vi "UserMgr-Window.vi"(7 "PwdMgr":refnum<class "PwdMgr.lvclass">, 8 "error in":errorcluster) -> (0 "error out":errorcluster)   [LabVIEW 2020, in "Login-UI.lvlib"]
uses:
  Login-UI.lvlib
  PwdMgr/PwdMgr.lvclass
  _Typedef/User-Info.ctl
  _Typedef/User-Role.ctl
  2fbc59fa-d6e3-46c3-98fb-aa3f40a50569.vi
  b49018c0-b0cc-4a1e-8c0a-6a6f7b5dc366.vi
  <userlib>/NEVSTOP-Programming-Palette/Configuration/ClusterCfgTable/Parse CfgTable(with DataName).vi
panel:
  in  "Table":i32(listbox)
  in  "编辑":bool
  in  "添加":bool
  in  "删除":bool
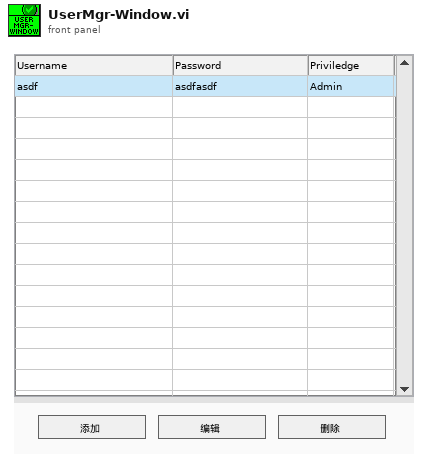
[diagram p1: front panel]
types:
  T1 = typedef "Login-UI.lvlib/User-Info.ctl" = cluster{"UserName":string, "Password":string, "Role":T2}
  T2 = typedef "Login-UI.lvlib/User-Role.ctl" = enum16{"INVALID", "Operator", "Engineer", "Admin", "Anonymous"}
  T3 = enum32{"Invalid", "Standard", "Closed", "Hidden", "Minimized", "Maximized"}
  T4 = enum32{"invalid app kind", "Development System", "Run Time System", "Student Edition", "Embedded LabVIEW", "Evaluation", "Custom"}
  T5 = cluster{"Core":cluster{"Current VI Reference":refnum<vi>, "Close Panel on Exit?":bool}, "Your Boolean data":bool, "Your string data":string, "Table Ref":refnum<vi>}
  T6 = cluster{"Current VI Reference":refnum<vi>, "Close Panel on Exit?":bool}
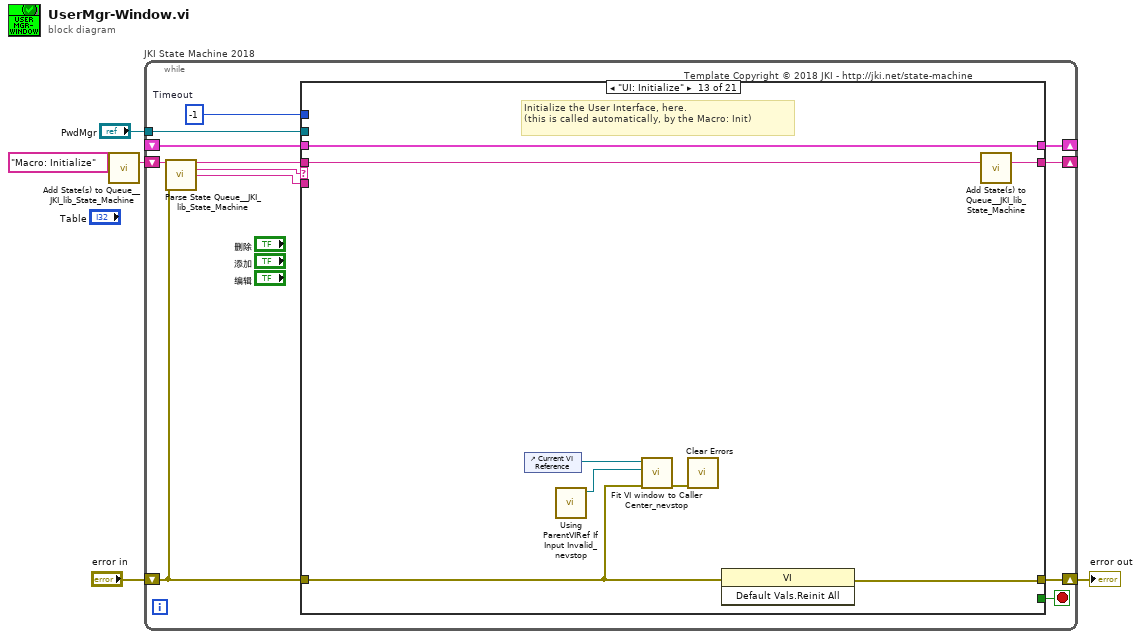
[diagram p0: block diagram]
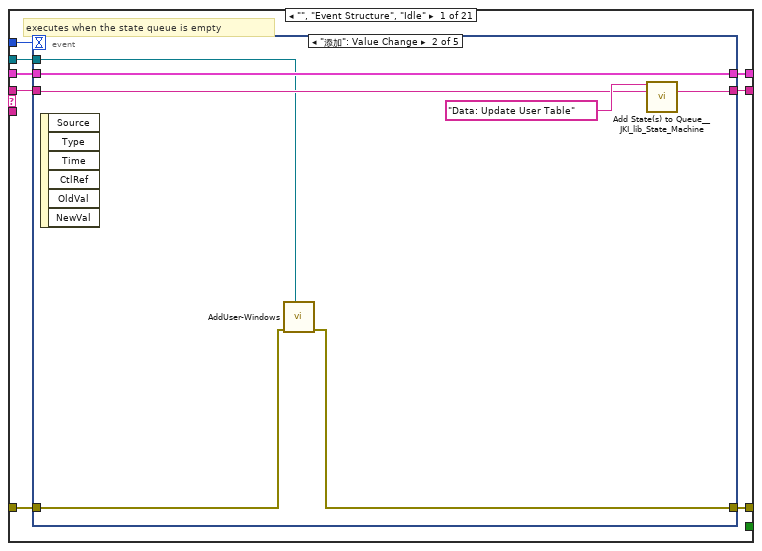
[diagram p2: hidden frame]
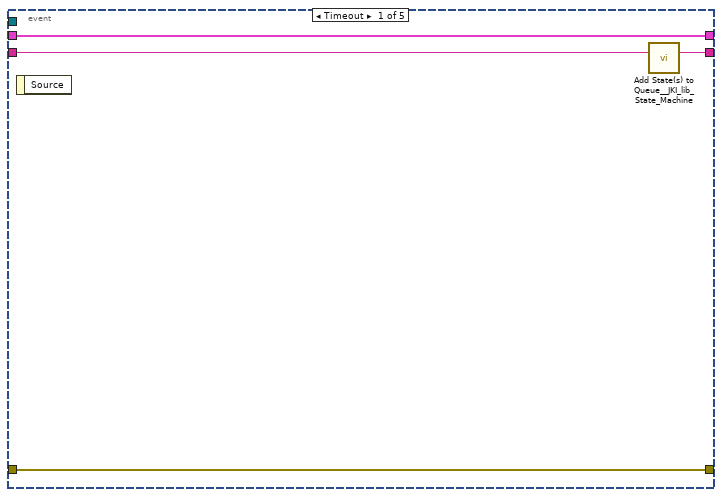
[diagram p3: hidden frame]
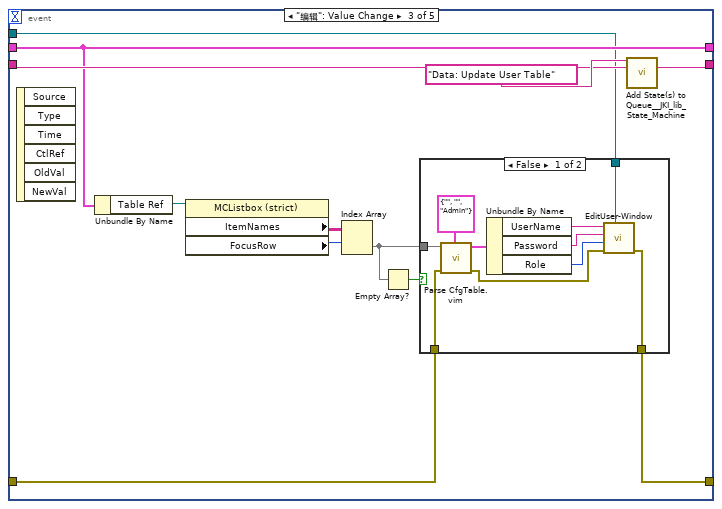
[diagram p4: hidden frame]
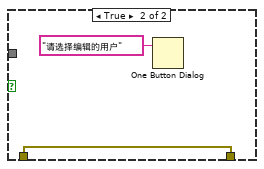
[diagram p5: hidden frame]
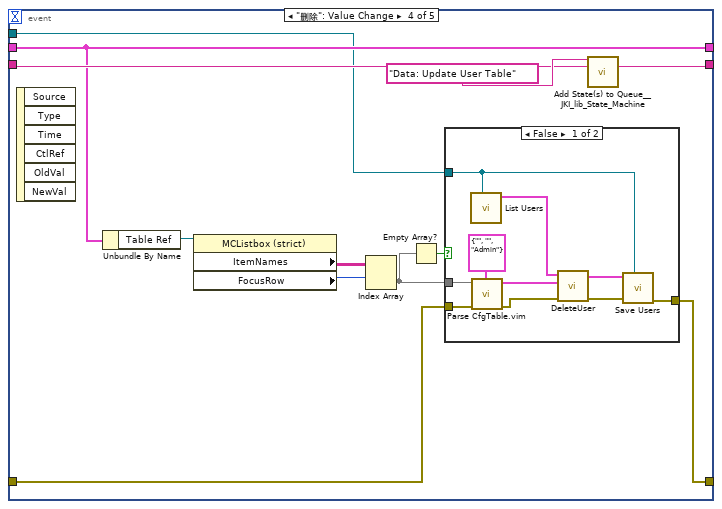
[diagram p6: hidden frame]
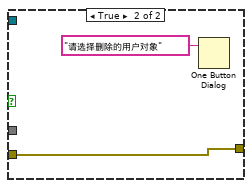
[diagram p7: hidden frame]
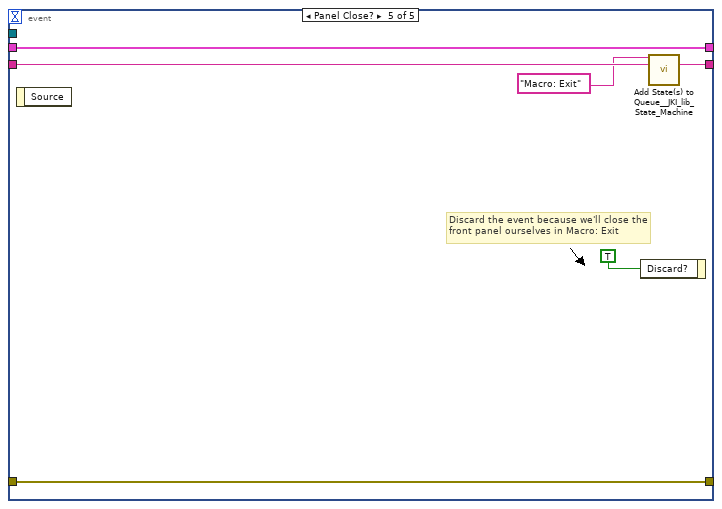
[diagram p8: hidden frame]
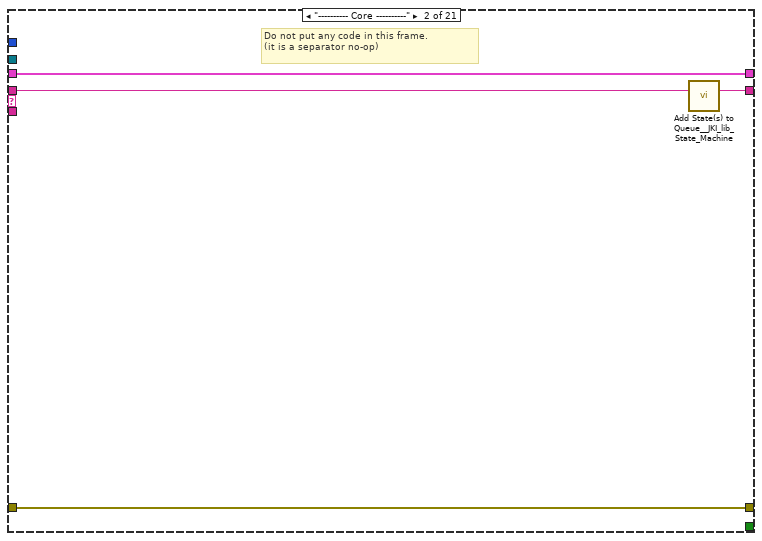
[diagram p9: hidden frame]
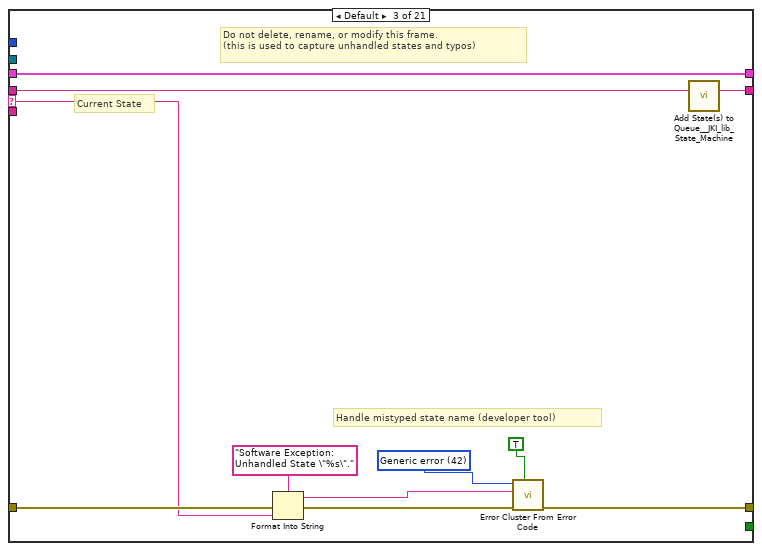
[diagram p10: hidden frame]
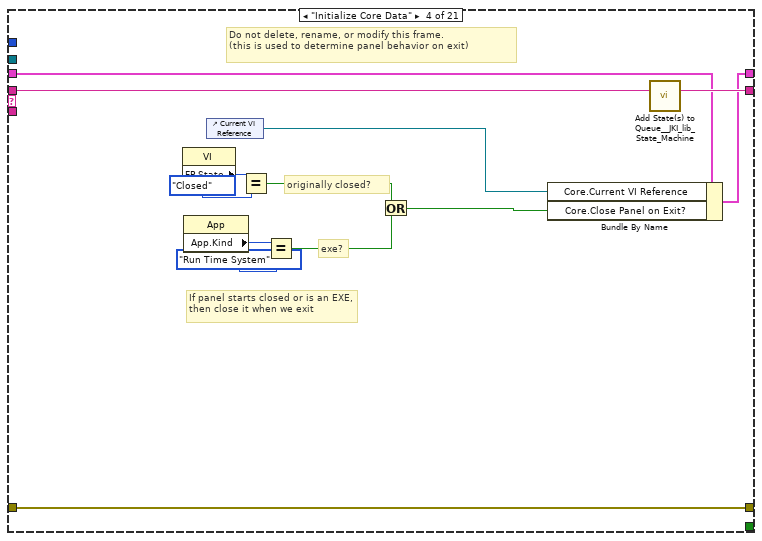
[diagram p11: hidden frame]
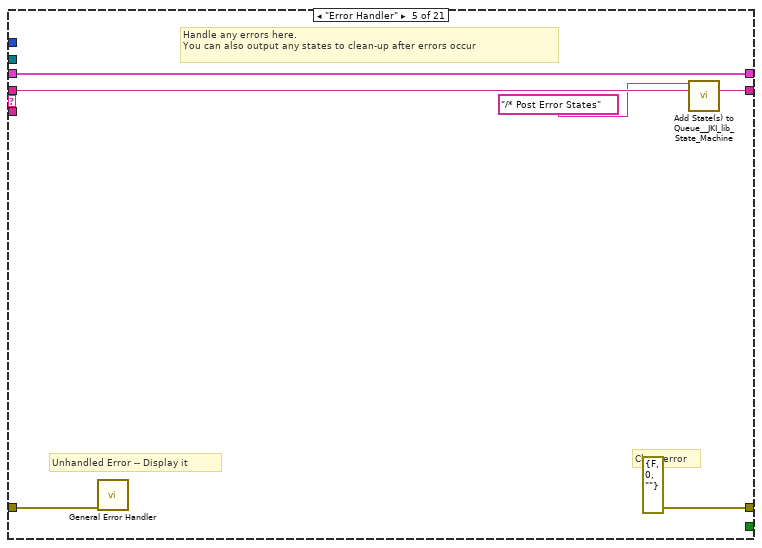
[diagram p12: hidden frame]
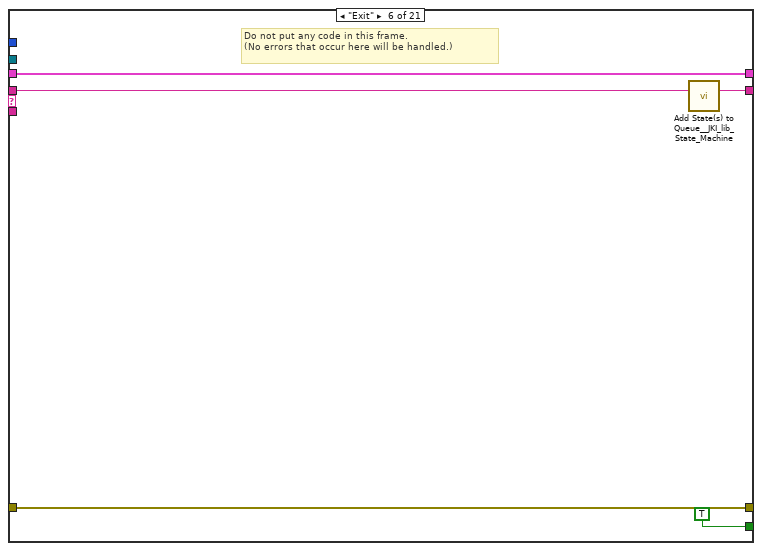
[diagram p13: hidden frame]
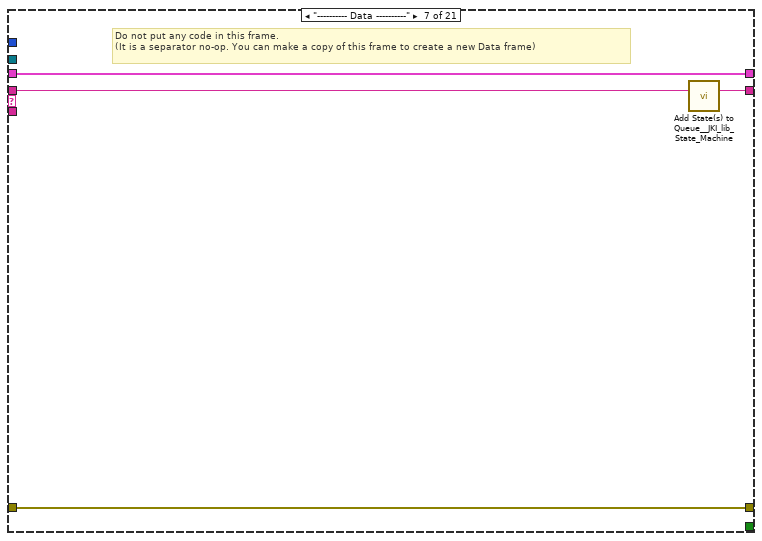
[diagram p14: hidden frame]
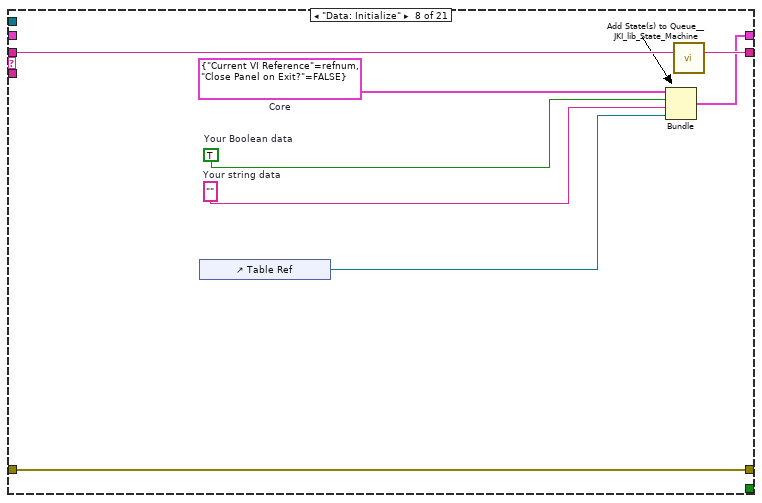
[diagram p15: hidden frame]
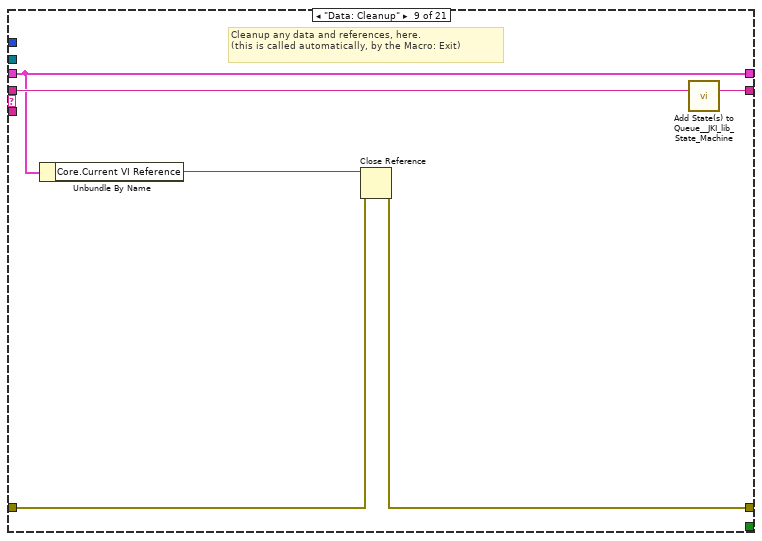
[diagram p16: hidden frame]
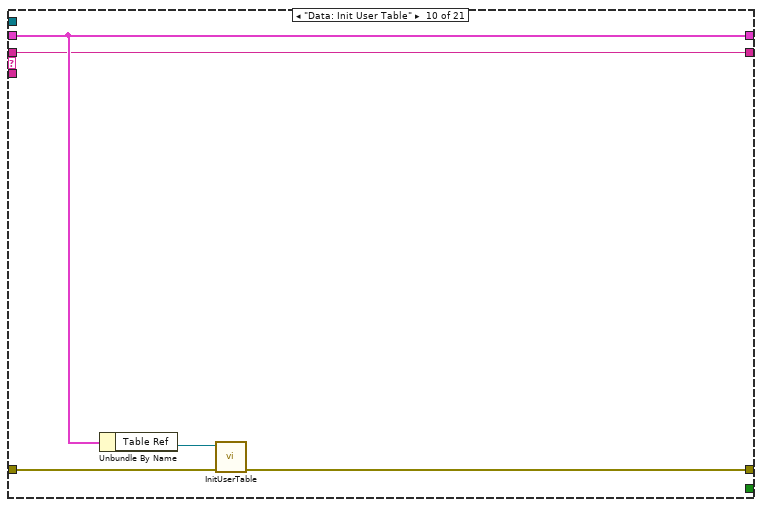
[diagram p17: hidden frame]
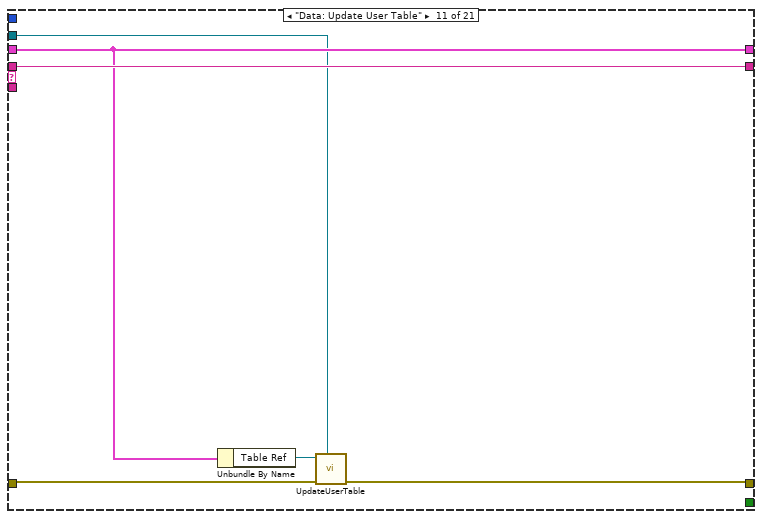
[diagram p18: hidden frame]
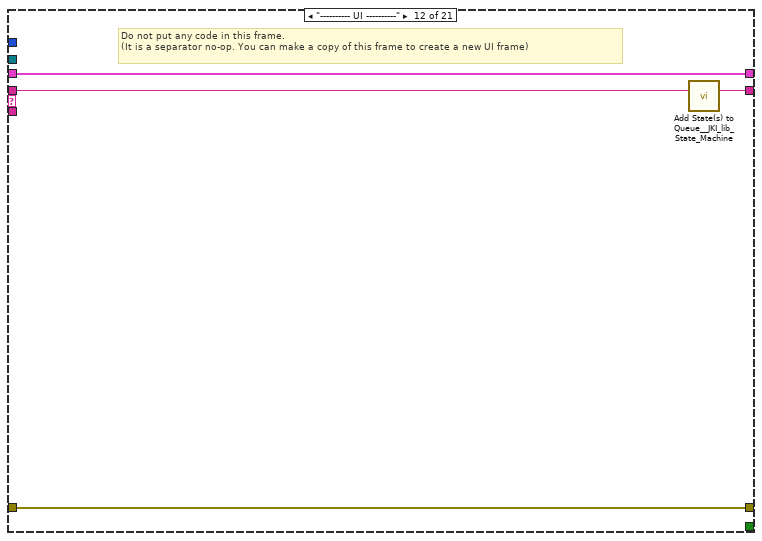
[diagram p19: hidden frame]
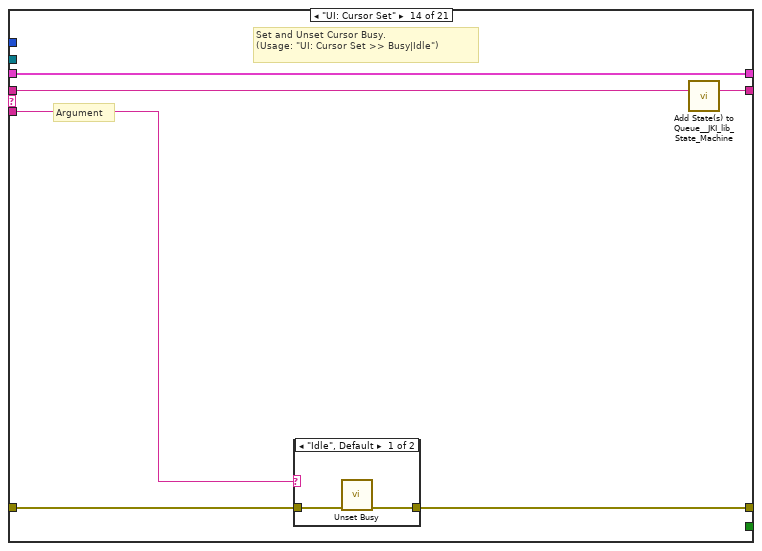
[diagram p20: hidden frame]
diagram:
  n1 = call <vilib>:"Add State(s) to Queue__JKI_lib_State_Machine.vi"("State(s) in (\"\")"="Macro: Initialize") -> ("States Out"=w5:string)  [unwired: 14 in]
  n2 = while "JKI State Machine 2018" {
    shift-right: [w10] -> _
    shift-left: _ -> [w9]
    shift-right: [w13] -> w2
    shift-left: "error in" -> [w7]
    shift-right: [w12] -> _
    shift-left: w5 -> [w14]
    tunnel: "PwdMgr" -> [w6]
    stop <- w11 stop-if-true
    w8 = -1  # Timeout
    # "Template Copyright © 2018 JKI - http://jki.net/state-machine"
    n3 = call <vilib>:"Parse State Queue__JKI_lib_State_Machine.vi"("State Queue"=w14, "Error In (no error)"=w7) -> ("Remaining States"=w16:string, "Current State"=w17:string, "Arguments"=w15:string)  [unwired: 11 in]
    n4 = case shown="\"UI: Initialize\"" w17 {
      selector: w17 -> [_ _ w95 _ _ _ _ _ _ _ _ _ _ _ _ _ _ _ _ _ _]
      tunnel: w16 -> [w25 w94 w99 w118 w124 w129 w133 w141 w147 w148 w155 w162 w170 w176 w187 w256 w261 w271 w275 w279 w283]
      tunnel: w15 -> [_ _ _ _ _ _ _ _ _ _ _ _ _ w171 w181 _ _ _ _ _ _]
      tunnel: w9 -> [w23 w91 w97 w111 w121 w127 w130 _ w142 w149 w154 w159 w168 w174 w183 w253 w258 w268 w272 w276 w280]
      tunnel: [w22 w92 w101 w115 errorcluster {"status"=FALSE, "code"=0, "source"=""} ("error out") w126 w131 w138 w143 w151 w157 w160 w166 w172 w184 w254 w259 w269 w273 w277 w281] -> w13
      tunnel: w7 -> [w21 w92 w100 w115 w120 w126 w131 w138 w144 w152 w158 w160 w167 w173 w185 w254 w259 w269 w273 w277 w281]
      tunnel: [w24 w93 w98 w117 w123 w128 w132 w140 w146 w148 w155 w161 w169 w175 w186 w255 w260 w270 w274 w278 w282] -> w12
      tunnel: [_ _ _ _ _ TRUE _ _ _ _ _ _ _ _ _ _ _ _ _ _ _] -> w11
      tunnel: [w20 w91 w97 w116 w121 w127 w130 w139 w142 w149 w154 w159 w168 w174 w183 w253 w258 w268 w272 w276 w280] -> w10
      tunnel: w8 -> [w19 _ _ _ _ _ _ _ _ _ _ _ _ _ _ _ _ _ _ _ _]
      tunnel: w6 -> [w18 _ _ _ _ _ _ _ _ _ w153 _ _ _ _ _ _ _ _ _ _]
      frame "", "Event Structure", "Idle" {
        # "executes when the state queue is empty"
        n5 = event shown="[1] \"添加\": Value Change" {
          selector: _ -> [_ _ _ _ _]
          dyn-events: _ -> [_ _ _ _ _]
          timeout: w19 -> [_ _ _ _ _]
          tunnel: w25 -> [w29 w34 w46 w70 w90]
          tunnel: [w28 w33 w47 w71 w89] -> w24
          tunnel: w23 -> [w26 w36 w45 w66 w87]
          tunnel: [w27 w31 w40 w62 w88] -> w22
          tunnel: w21 -> [w27 w32 w41 w63 w88]
          tunnel: [w26 w36 w45 w66 w87] -> w20
          tunnel: w18 -> [_ w30 w37 w61 _]
          event Timeout {
            n6 = event-data() -> ()  [unwired: 1 in, 1 out]
            n7 = call <vilib>:"Add State(s) to Queue__JKI_lib_State_Machine.vi"("State(s) in (\"\")"=w29) -> ("States Out"=w28:string)  [unwired: 14 in]
          }
          event "添加": Value Change {
            n8 = event-data() -> ()  [unwired: 1 in, 6 out]
            n9 = call "AddUser-Windows.vi"("Login-UI.lvlib:PwdMgr.lvclass"=w30, "error in"=w32) -> ("error out"=w31:errorcluster)  [unwired: 9 in]
            n10 = call <vilib>:"Add State(s) to Queue__JKI_lib_State_Machine.vi"("State(s) in Front (\"\")"="Data: Update User Table", "State(s) in (\"\")"=w34) -> ("States Out"=w33:string)  [unwired: 13 in]
          }
          event "编辑": Value Change {
            n11 = event-data() -> ()  [unwired: 1 in, 6 out]
            n12 = Unbundle By Name(w45) -> ("Table Ref"=w44:refnum<vi>)
            n13 = property class="MCListbox (strict)"(reference=w44) -> ("ItemNames"=w43:string[][], "FocusRow"=w42:i32)  [unwired: 1 in, 2 out]
            n14 = Index Array(array=w43, index (row)=w42) -> (element=w38:string[])  [unwired: 1 in]
            n15 = Empty Array?(array=w38) -> (empty?=w39:bool)
            n16 = case shown="False" w39 {
              tunnel: w38 -> [w58 _]
              tunnel: w41 -> [w52 w59]
              tunnel: [w50 w59] -> w40
              tunnel: w37 -> [w49 _]
              frame False {
                n17 = call "Parse CfgTable.vim"("Cluster Configuration Typedef"=T1 {"UserName"="", "Password"="", "Role"=enum."Admin"} ("Cluster"), "error in (no error)"=w52, "CfgTable Row"=w58) -> ("error out"=w51:errorcluster, "Cluster Configuration Out"=w56:T1)  [unwired: 7 in]
                n18 = Unbundle By Name(w56) -> ("UserName"=w55:string, "Password"=w54:string, "Role"=w53:T2)
                n19 = call "EditUser-Window.vi"("Login-UI.lvlib:PwdMgr.lvclass"=w49, "error in"=w51, "权  限"=w53, "密  码"=w54, "用户名"=w55) -> ("error out"=w50:errorcluster)  [unwired: 6 in]
              }
              frame True {
                n20 = One Button Dialog(message="请选择编辑的用户") -> ()  [unwired: 1 in, 1 out]
              }
            }
            n21 = call <vilib>:"Add State(s) to Queue__JKI_lib_State_Machine.vi"("State(s) in Front (\"\")"="Data: Update User Table", "State(s) in (\"\")"=w46) -> ("States Out"=w47:string)  [unwired: 13 in]
          }
          event "删除": Value Change {
            n22 = event-data() -> ()  [unwired: 1 in, 6 out]
            n23 = Unbundle By Name(w66) -> ("Table Ref"=w69:refnum<vi>)
            n24 = property class="MCListbox (strict)"(reference=w69) -> ("ItemNames"=w68:string[][], "FocusRow"=w67:i32)  [unwired: 1 in, 2 out]
            n25 = Index Array(array=w68, index (row)=w67) -> (element=w64:string[])  [unwired: 1 in]
            n26 = Empty Array?(array=w64) -> (empty?=w65:bool)
            n27 = case shown="False" w65 {
              tunnel: w64 -> [w82 _]
              tunnel: w63 -> [w75 w83]
              tunnel: [w74 w83] -> w62
              tunnel: w61 -> [w73 _]
              frame False {
                n28 = call-dynamic "List Users.vi"("PwdMgr in"=w73) -> ("Array"=w80:T1[])  [unwired: 9 in, 1 out]
                n29 = call "Parse CfgTable.vim"("Cluster Configuration Typedef"=T1 {"UserName"="", "Password"="", "Role"=enum."Admin"} ("Cluster"), "error in (no error)"=w75, "CfgTable Row"=w82) -> ("error out"=w76:errorcluster, "Cluster Configuration Out"=w79:T1)  [unwired: 7 in]
                n30 = call "DeleteUser.vi"("error in"=w76, "User"=w79, "User List"=w80) -> ("error out"=w77:errorcluster, "User List"=w78:T1[])  [unwired: 7 in]
                n31 = call-dynamic "Save Users.vi"("PwdMgr in"=w73, "error in (no error)"=w77, "Array"=w78) -> ("error out"=w74:errorcluster)  [unwired: 8 in]
              }
              frame True {
                n32 = One Button Dialog(message="请选择删除的用户对象") -> ()  [unwired: 1 in, 1 out]
              }
            }
            n33 = call <vilib>:"Add State(s) to Queue__JKI_lib_State_Machine.vi"("State(s) in Front (\"\")"="Data: Update User Table", "State(s) in (\"\")"=w70) -> ("States Out"=w71:string)  [unwired: 13 in]
          }
          event Panel Close? {
            # "Discard the event because we'll close the front panel ourselves in Macro: Exit"
            n34 = event-data() -> ()  [unwired: 1 in, 1 out]
            n35 = event-data("Discard?"=TRUE) -> ()  [unwired: 1 in, 1 out]
            n36 = call <vilib>:"Add State(s) to Queue__JKI_lib_State_Machine.vi"("State(s) in Front (\"\")"="Macro: Exit", "State(s) in (\"\")"=w90) -> ("States Out"=w89:string)  [unwired: 13 in]
          }
        }
      }
      frame "---------- Core ----------" {
        # "Do not put any code in this frame.\n(it is a separator no-op)"
        n37 = call <vilib>:"Add State(s) to Queue__JKI_lib_State_Machine.vi"("State(s) in (\"\")"=w94) -> ("States Out"=w93:string)  [unwired: 14 in]
      }
      frame Default {
        w104 = 42 items=["No error", "Argument error", "Memory is full", "Out of zone", "End of file", "File already open", "Generic file I/O error", "File not found", "File permission error", "Disk is full", "Duplicate path", "Too many files open", "System feature not enabled", "Resource file not found", "Cannot add resource", "Resource not found", "Image not found", "Image memory error", "Pen does not exist", "Config type invalid", "Config token not found", "Config parse error", "Config memory error", "Bad external code format", "Bad external code offset", "External code not present", "Null window", "Destroy window error", "Null menu", "Print aborted", "Bad print record", "Print driver error", "Windows error during printing", "Memory error during printing", "Print dialog error", "Generic print error", "Invalid device refnum", "Device not found", "Device parameter error", "Device unit error", "Cannot open device", "Device call aborted", "Generic error", "Cancelled by user", "Object ID too low", "Object ID too high", "Object not in heap", "Unknown heap", "Unknown object (invalid DefProc)", "Unknown object (DefProc not in table)", "Message out of range", "Invalid (null) method", "Unknown message", "Manager call not supported", "Bad address", "Network operation in progress", "Network operation timed out", "Connection is busy", "Network attribute not supported", "Network error", "Address in use", "System out of memory", "Connection aborted", "Connection refused", "Not connected", "Already connected", "Connection closed", "Initialization error (interapplication manager)", "Bad occurrence", "Wait on unbound occurrence handler", "Occurrence queue overflow", "Datalog type conflict", "Unused", "Unrecognized type (interapplication manager)", "Memory corrupt", "Failed to make temporary DLL", "Old CIN version", "Drag socket not found", "Failed to load drop-object", "Failed to register OLE object", "Failed to release OLE object", "Format specifier type mismatch", "Unknown format specifier", "Too few format specifiers", "Too many format specifiers", "Scan failed", "Newer CIN version", "Error converting to variant", "Runtime menu error", "Password tampered", "Variant attribute not found", "Incompatible variant data type", "Event data is not available", "Event Store is not present", "Occurrence is not found", "Event Queue is not created", "Event info is not available", "Refnum passed is NULL", "Error retrieving Class GUID", "Error retrieving CoClass GUID", "Error retrieving TypeLib GUID.", "Bad built application magic bytes.", "Specific driver is different from the specific driver associated with the Logical Name.", "There is no session opened to the class driver.", "Max Error", "MAX - Error with config objects", "MAX - Error loading configuration", "MAX - Group not supported"]
        # "Current State"
        # "Do not delete, rename, or modify this frame.\n(this is used to capture unhandled states and typos)"
        # "Handle mistyped state name (developer tool)"
        n38 = Format Into String(format string="Software Exception: Unhandled State \"%s\"." ("message"), error in=w100, w95) -> (resulting string=w103:string, error out=w102:errorcluster)  [unwired: 1 in]
        n39 = call <vilib>:"Error Cluster From Error Code.vi"("show call chain? (False)"=TRUE, "error in (no error)"=w102, "error message (\"\")"=w103, "error code (0)"=w104) -> ("error out"=w101:errorcluster)  [unwired: 5 in]
        n40 = call <vilib>:"Add State(s) to Queue__JKI_lib_State_Machine.vi"("State(s) in (\"\")"=w99) -> ("States Out"=w98:string)  [unwired: 14 in]
      }
      frame "Initialize Core Data" {
        # "Do not delete, rename, or modify this frame.\n(this is used to determine panel behavior on exit)"
        # "originally closed?"
        # "exe?"
        # "If panel starts closed or is an EXE, then close it when we exit"
        n41 = property class="VI"() -> ("FP.State"=w108:T3)  [unwired: 2 in, 2 out]
        n42 = property class="App"() -> ("App.Kind"=w114:T4)  [unwired: 2 in, 2 out]
        n43 = control-ref of="Current VI Reference"() -> (w109:refnum<vi>)
        n44 = Equal?(x=w108, y=T3."Closed" ("Front Panel Window:State")) -> (x = y?=w106:bool)
        n45 = Equal?(x=w114, y=T4."Run Time System" ("Application:Kind")) -> (x = y?=w112:bool)
        n46 = Or(x=w106, y=w112) -> (x .or. y?=w110:bool)
        n47 = Bundle By Name(cluster=w111, "Core.Current VI Reference"=w109, "Core.Close Panel on Exit?"=w110) -> (w116:T5)
        n48 = call <vilib>:"Add State(s) to Queue__JKI_lib_State_Machine.vi"("State(s) in (\"\")"=w118) -> ("States Out"=w117:string)  [unwired: 14 in]
      }
      frame "Error Handler" {
        # "Unhandled Error -- Display it"
        # "Handle any errors here.\nYou can also output any states to clean-up after errors occur"
        # "Clear error"
        n49 = call <vilib>:"General Error Handler.vi"("error in (no error)"=w120) -> ()  [unwired: 10 in, 5 out]
        n50 = call <vilib>:"Add State(s) to Queue__JKI_lib_State_Machine.vi"("State(s) in Front (\"\")"="/* Post Error States", "State(s) in (\"\")"=w124) -> ("States Out"=w123:string)  [unwired: 13 in]
      }
      frame "Exit" {
        # "Do not put any code in this frame.\n(No errors that occur here will be handled.)"
        n51 = call <vilib>:"Add State(s) to Queue__JKI_lib_State_Machine.vi"("State(s) in (\"\")"=w129) -> ("States Out"=w128:string)  [unwired: 14 in]
      }
      frame "---------- Data ----------" {
        # "Do not put any code in this frame.\n(It is a separator no-op. You can make a copy of this frame to create a new Data frame)"
        n52 = call <vilib>:"Add State(s) to Queue__JKI_lib_State_Machine.vi"("State(s) in (\"\")"=w133) -> ("States Out"=w132:string)  [unwired: 14 in]
      }
      frame "Data: Initialize" {
        w135 = T6 {"Current VI Reference"=refnum, "Close Panel on Exit?"=FALSE}  # Core
        w137 = TRUE  # Your Boolean data
        w136 = ""  # Your string data
        n53 = control-ref of="Table Ref"() -> (w134:refnum<vi>)
        n54 = Bundle("Core"=w135, "Your Boolean data"=w137, "Your string data"=w136, "Table Ref"=w134) -> (w139:T5)  [unwired: 1 in]
        n55 = call <vilib>:"Add State(s) to Queue__JKI_lib_State_Machine.vi"("State(s) in (\"\")"=w141) -> ("States Out"=w140:string)  [unwired: 14 in]
      }
      frame "Data: Cleanup" {
        # "Cleanup any data and references, here.\n(this is called automatically, by the Macro: Exit)"
        n56 = Unbundle By Name(w142) -> ("Core.Current VI Reference"=w145:refnum<vi>)
        n57 = Close Reference(reference=w145, error in (no error)=w144) -> (error out=w143:errorcluster)
        n58 = call <vilib>:"Add State(s) to Queue__JKI_lib_State_Machine.vi"("State(s) in (\"\")"=w147) -> ("States Out"=w146:string)  [unwired: 14 in]
      }
      frame "Data: Init User Table" {
        n59 = Unbundle By Name(w149) -> ("Table Ref"=w150:refnum<vi>)
        n60 = call "InitUserTable.vi"("Error in"=w152, "User Table"=w150) -> ("error out"=w151:errorcluster)  [unwired: 9 in]
      }
      frame "Data: Update User Table" {
        n61 = Unbundle By Name(w154) -> ("Table Ref"=w156:refnum<vi>)
        n62 = call "UpdateUserTable.vi"("Login-UI.lvlib:PwdMgr.lvclass"=w153, "Error in"=w158, "User Table"=w156) -> ("error out"=w157:errorcluster)  [unwired: 8 in]
      }
      frame "---------- UI ----------" {
        # "Do not put any code in this frame.\n(It is a separator no-op. You can make a copy of this frame to create a new UI frame)"
        n63 = call <vilib>:"Add State(s) to Queue__JKI_lib_State_Machine.vi"("State(s) in (\"\")"=w162) -> ("States Out"=w161:string)  [unwired: 14 in]
      }
      frame "UI: Initialize" {
        # "Initialize the User Interface, here.\n(this is called automatically, by the Macro: Init)"
        n64 = control-ref of="Current VI Reference"() -> (w164:refnum<vi>)
        n65 = call <userlib>:"Using ParentVIRef If Input Invalid_nevstop.vi"() -> ("VI Ref"=w163:refnum<vi>)  [unwired: 6 in, 1 out]
        n66 = call <userlib>:"Fit VI window to Caller Center_nevstop.vi"("Error In"=w167, "Background VI Ref (Callee's Caller)"=w163, "VI Ref (calling VI)"=w164) -> ("Error Out"=w165:errorcluster)  [unwired: 3 in, 1 out]
        n67 = call <vilib>:"Clear Errors.vi"("error in (no error)"=w165) -> ()  [unwired: 5 in, 2 out]
        n68 = invoke class="VI" method="Default Vals.Reinit All"(error in=w167) -> (error out=w166:errorcluster)  [unwired: 2 in, 2 out]
        n69 = call <vilib>:"Add State(s) to Queue__JKI_lib_State_Machine.vi"("State(s) in (\"\")"=w170) -> ("States Out"=w169:string)  [unwired: 14 in]
      }
      frame "UI: Cursor Set" {
        # "Argument"
        # "Set and Unset Cursor Busy.\n(Usage: \"UI: Cursor Set >> Busy|Idle\")"
        n70 = case shown="\"Idle\", Default" w171 {
          tunnel: w173 -> [w178 w180]
          tunnel: [w177 w179] -> w172
          frame "Idle", Default {
            n71 = call <vilib>:"Unset Busy.vi"("error in (no error)"=w178) -> ("error out"=w177:errorcluster)  [unwired: 10 in]
          }
          frame "Busy" {
            n72 = call <vilib>:"Set Busy.vi"("error in (no error)"=w180) -> ("error out"=w179:errorcluster)  [unwired: 9 in, 1 out]
          }
        }
        n73 = call <vilib>:"Add State(s) to Queue__JKI_lib_State_Machine.vi"("State(s) in (\"\")"=w176) -> ("States Out"=w175:string)  [unwired: 14 in]
      }
      frame "UI: Front Panel State" {
        # "Argument"
        # "Set Front Panel Open or Closed\n(Usage: \"UI: Front Panel State >> Open|Close\")"
        n74 = Unbundle By Name(w183) -> ("Core.Current VI Reference"=w182:refnum<vi>)
        n75 = case shown="\"Minimize\", \"Minimized\"" w181 {
          tunnel: w185 -> [w193 w208 w219 w232 w245]
          tunnel: [w195 w209 w221 w234 w247] -> w184
          tunnel: w182 -> [w194 w206 w220 w233 w246]
          frame "Open", "Standard", Default {
            w188 = T3."Standard" ("State")
            n76 = property class="VI"(reference=w194, error in=w193) -> (reference out=w191:refnum<vi>, error out=w192:errorcluster, "FP.State"=w190:T3)
            n77 = Not Equal?(x=w190, y=w188) -> (x != y?=w189:bool)
            n78 = case shown="True" w189 {
              tunnel: [w199 w201] -> w195
              tunnel: w192 -> [w198 w201]
              tunnel: w191 -> [w197 _]
              tunnel: w188 -> [w196 _]
              frame True {
                n79 = invoke class="VI" method="FP.Open"(reference=w197, error in=w198, "Activate"=TRUE, "State"=w196) -> (error out=w199:errorcluster)  [unwired: 1 in, 4 out]
              }
              frame False {
              }
            }
          }
          frame "Close", "Closed" {
            n80 = property class="VI"(reference=w206, error in=w208) -> (reference out=w205:refnum<vi>, error out=w207:errorcluster, "FP.State"=w203:T3)
            n81 = Not Equal?(x=w203, y=T3."Closed" ("Front Panel Window:State")) -> (x != y?=w202:bool)
            n82 = case shown="True" w202 {
              tunnel: [w210 w213] -> w209
              tunnel: w207 -> [w210 w212]
              tunnel: w205 -> [_ w211]
              frame False {
              }
              frame True {
                n83 = invoke class="VI" method="FP.Close"(reference=w211, error in=w212) -> (error out=w213:errorcluster)  [unwired: 1 in, 2 out]
              }
            }
          }
          frame "Hidden", "Hide" {
            w214 = T3."Hidden" ("State")
            n84 = property class="VI"(reference=w220, error in=w219) -> (reference out=w217:refnum<vi>, error out=w218:errorcluster, "FP.State"=w216:T3)
            n85 = Not Equal?(x=w216, y=w214) -> (x != y?=w215:bool)
            n86 = case shown="True" w215 {
              tunnel: [w225 w226] -> w221
              tunnel: w218 -> [w224 w226]
              tunnel: w217 -> [w223 _]
              tunnel: w214 -> [w222 _]
              frame True {
                n87 = invoke class="VI" method="FP.Open"(reference=w223, error in=w224, "State"=w222) -> (error out=w225:errorcluster)  [unwired: 2 in, 4 out]
              }
              frame False {
              }
            }
          }
          frame "Minimize", "Minimized" {
            w227 = T3."Minimized" ("State")
            n88 = property class="VI"(reference=w233, error in=w232) -> (reference out=w230:refnum<vi>, error out=w231:errorcluster, "FP.State"=w229:T3)
            n89 = Not Equal?(x=w229, y=w227) -> (x != y?=w228:bool)
            n90 = case shown="True" w228 {
              tunnel: [w238 w239] -> w234
              tunnel: w231 -> [w237 w239]
              tunnel: w230 -> [w236 _]
              tunnel: w227 -> [w235 _]
              frame True {
                n91 = invoke class="VI" method="FP.Open"(reference=w236, error in=w237, "State"=w235) -> (error out=w238:errorcluster)  [unwired: 2 in, 4 out]
              }
              frame False {
              }
            }
          }
          frame "Maximize", "Maximized" {
            w240 = T3."Maximized" ("State")
            n92 = property class="VI"(reference=w246, error in=w245) -> (reference out=w243:refnum<vi>, error out=w244:errorcluster, "FP.State"=w242:T3)
            n93 = Not Equal?(x=w242, y=w240) -> (x != y?=w241:bool)
            n94 = case shown="True" w241 {
              tunnel: [w251 w252] -> w247
              tunnel: w244 -> [w250 w252]
              tunnel: w243 -> [w249 _]
              tunnel: w240 -> [w248 _]
              frame True {
                n95 = invoke class="VI" method="FP.Open"(reference=w249, error in=w250, "State"=w248) -> (error out=w251:errorcluster)  [unwired: 2 in, 4 out]
              }
              frame False {
              }
            }
          }
        }
        n96 = call <vilib>:"Add State(s) to Queue__JKI_lib_State_Machine.vi"("State(s) in (\"\")"=w187) -> ("States Out"=w186:string)  [unwired: 14 in]
      }
      frame "---------- Macro ----------" {
        # "Do not put any code in this frame.\n(It is a separator no-op. You can make a copy of this frame to create a new Macro frame)"
        n97 = call <vilib>:"Add State(s) to Queue__JKI_lib_State_Machine.vi"("State(s) in (\"\")"=w256) -> ("States Out"=w255:string)  [unwired: 14 in]
      }
      frame "Macro: Initialize" {
        w257 = "Data: Initialize\nInitialize Core Data\nUI: Initialize\nUI: Front Panel State >> Open\nData: Init User Table\nData: Update User Table"  # Data: Initialize Initialize Core Data UI: Initialize UI: Front Panel State >> Open Data: Init User Table Data: Update User Table
        # "Initialization Macro\n(This is called once, when the VI starts)"
        n98 = call <vilib>:"Add State(s) to Queue__JKI_lib_State_Machine.vi"("State(s) in Front (\"\")"=w257, "State(s) in (\"\")"=w261) -> ("States Out"=w260:string)  [unwired: 13 in]
      }
      frame "Macro: Exit" {
        # "Exit Macro\n(This is called once, when the VI exits)"
        n99 = Unbundle By Name(w268) -> ("Core.Close Panel on Exit?"=w267:bool)
        n100 = Select(t="UI: Front Panel State >> Close", s=w267, f="") -> (s? t:f=w264:string)
        n101 = call <vilib>:"Add State(s) to Queue__JKI_lib_State_Machine.vi"("State(s) in (\"\")"=w264, "State(s) at Back (\"\")"="Data: Cleanup\nExit") -> ("States Out"=w262:string)  [unwired: 13 in]
        n102 = call <vilib>:"Add State(s) to Queue__JKI_lib_State_Machine.vi"("State(s) in Front (\"\")"=w262, "State(s) in (\"\")"=w271) -> ("States Out"=w270:string)  [unwired: 13 in]
      }
      frame "---------- New Category ----------" {
        # "Template Separator\n(You can make a copy of, or modify, this frame)"
        n103 = call <vilib>:"Add State(s) to Queue__JKI_lib_State_Machine.vi"("State(s) in (\"\")"=w275) -> ("States Out"=w274:string)  [unwired: 14 in]
      }
      frame "New Category: 1" {
        # "Your code here.\n(You can make a copy of, or modify, this frame)"
        n104 = call <vilib>:"Add State(s) to Queue__JKI_lib_State_Machine.vi"("State(s) in (\"\")"=w279) -> ("States Out"=w278:string)  [unwired: 14 in]
      }
      frame "New Category: 2" {
        # "Your code here.\n(You can make a copy of, or modify, this frame)"
        n105 = call <vilib>:"Add State(s) to Queue__JKI_lib_State_Machine.vi"("State(s) in (\"\")"=w283) -> ("States Out"=w282:string)  [unwired: 14 in]
      }
    }
  }
  "error out" <- w2
